vi "Test FIFO Space Check with Roll Over.vi"() -> ()   [LabVIEW 2021]
uses:
  <vilib>/CIF Foundation/CIF Utilities/Boolean/Boolean/Latch.vi
  CIF_NI_CIPC.lvlib
panel:
  out "error out":errorcluster
  out "pass":bool
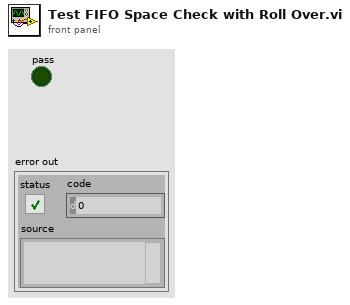
[diagram p1: front panel]
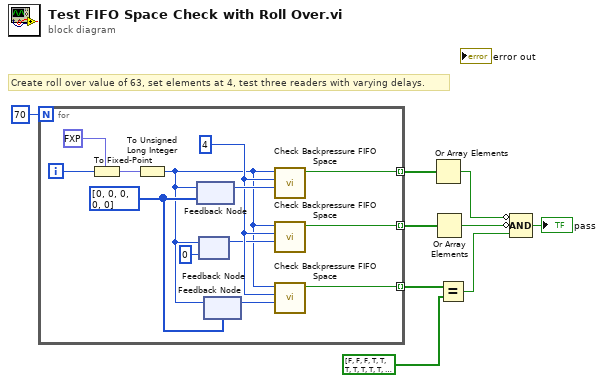
[diagram p0: block diagram]
diagram:
  # "Create roll over value of 63, set elements at 4, test three readers with varying delays."
  n1 = for {
    N: 70 -> [_]
    tunnel: [w18] -> w8 mode=indexing
    tunnel: [w17] -> w7 mode=indexing
    tunnel: [w14] -> w3 mode=indexing
    i -> [w22]
    w16 = u32 4 ("Elements")
    w15 = u32[] [0, 0, 0, 0, 0]
    n2 = To Fixed-Point(fixed-point type=fxp<+,6,6> 0.0, number=w22) -> (fixed-point=w20:fxp<+,6,6>)
    n3 = To Unsigned Long Integer(number=w20) -> (unsigned 32bit integer=w11:u32)
    n4 = feedback-in #1(w11) -> ()
    n5 = feedback #1(w15) -> (w19:u32)
    n6 = feedback #2(u32 0) -> (w12:u32)
    n7 = feedback-in #2(w11) -> ()
    n8 = feedback #3(w15) -> (w13:u32)
    n9 = feedback-in #3(w11) -> ()
    n10 = call "Check Backpressure FIFO Space.vi"("Read Pos (from BP)"=w19, "Elements"=w16, "Write Pos"=w11) -> ("Full"=w18:bool)  [unwired: 8 in]
    n11 = call "Check Backpressure FIFO Space.vi"("Read Pos (from BP)"=w12, "Elements"=w16, "Write Pos"=w11) -> ("Full"=w17:bool)  [unwired: 8 in]
    n12 = call "Check Backpressure FIFO Space.vi"("Read Pos (from BP)"=w13, "Elements"=w16, "Write Pos"=w11) -> ("Full"=w14:bool)  [unwired: 8 in]
  }
  n13 = Or Array Elements(Boolean array=w8) -> (logical OR=w6:bool)
  n14 = Or Array Elements(Boolean array=w7) -> (logical OR=w5:bool)
  n15 = Equal?(x=w3, y=bool[] [FALSE, FALSE, FALSE, TRUE, TRUE, TRUE, TRUE, TRUE, TRUE, TRUE, TRUE, TRUE, TRUE, TRUE, TRUE, TRUE, TRUE, TRUE, TRUE, TRUE, TRUE, TRUE, TRUE, TRUE, TRUE, TRUE, TRUE, TRUE, TRUE, TRUE, TRUE, TRUE, TRUE, TRUE, TRUE, TRUE, TRUE, TRUE, TRUE, TRUE, TRUE, TRUE, TRUE, TRUE, TRUE, TRUE, TRUE, TRUE, TRUE, TRUE, TRUE, TRUE, TRUE, TRUE, TRUE, TRUE, TRUE, TRUE, TRUE, TRUE, TRUE, TRUE, TRUE, TRUE, TRUE, TRUE, TRUE, TRUE, TRUE, TRUE] ("Array 4")) -> (x = y?=w2:bool)
  n16 = Compound Arithmetic op=AND(invert w6, invert w5, w2) -> (→"pass":bool)
